vi "motor test 001.vi"() -> ()   [LabVIEW 2019]
uses:
  <vilib>/Platform/TimedLoop/XDataNode/timing_clust.ctl
  <vilib>/Platform/TimedLoop/XDataNode/nitl_modes.ctl
  <vilib>/Platform/TimedLoop/XDataNode/wakeup.ctl
  low level/motor/motor.lvclass
  <vilib>/platform/TimedLoop/XDataNode/XDataNode.xnode
  <vilib>/Platform/TimedLoop/XDataNode/XDNodeRunTimeDep.lvlib
panel:
  in  "Stop":bool
  out "error out":errorcluster
  in  "Error In":errorcluster
  in  "Vertical Pointer Slide":dbl(slide) scale=-125.0..125.0
  in  "reset":bool
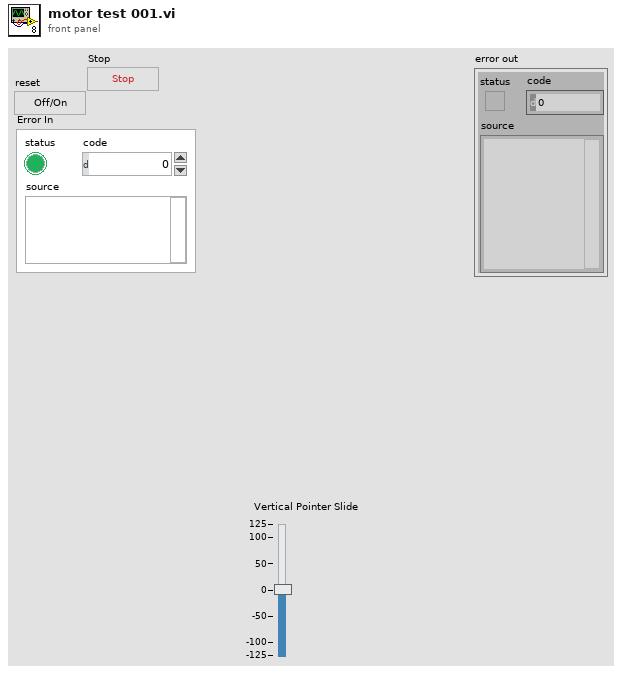
[diagram p1: front panel]
types:
  T1 = typedef "XDNodeRunTimeDep.lvlib/timing_clust.ctl" = cluster{"Expected End [f-1]":u64, "Actual End [f-1]":u64, "Finished Late? [f-1]":bool, "Expected End [i-1]":u64, "Actual End [i-1]":u64, "Finished Late? [i-1]":bool, "Expected Start [i]":u64, "Actual Start [i]":u64, "Expected Start [f]":u64, "Actual Start [f]":u64, "Source Name":string, "Structure Name":string, "Period":i64, "Deadline":i64, "Offset":i64, "Start":i64, "Priority":i32, "Timeout":i32, "Mode":T2, "Wakeup Reason":T3, "Error":errorcluster, "Source Type":string, "Secondary Source Type":string, "Global End Time":u64, "Global Start Time":u64, "Frame Duration":u64, "Iteration Duration":u64, "Assigned CPU":i32, "I/O Scan Engine Mode":u32}
  T2 = typedef "XDNodeRunTimeDep.lvlib/nitl_modes.ctl" = enum32{"No Change", "Process missed periods, maintain original phase", "Discard missed periods, maintain original phase", "Process missed periods, ignore original phase", "Discard missed periods, ignore original phase"}
  T3 = typedef "XDNodeRunTimeDep.lvlib/wakeup.ctl" = enum32{"Normal", "Aborted", "Asynchronous wakeup", "Timing source error", "Timed loop error", "Timeout"}
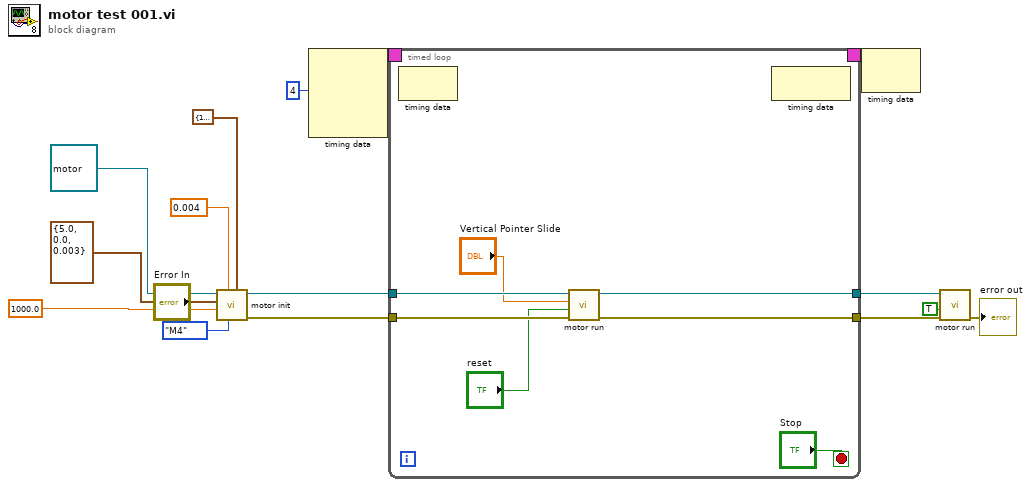
[diagram p0: block diagram]
diagram:
  n1 = call "motor init.vi"("encoder"=cluster{"encoder PPR":dbl, "gear ratio":dbl} {"encoder PPR"=16.0, "gear ratio"=64.0}, "motor  ?"=enum16{"M1", "M2", "M3", "M4"}."M4", "dt"=0.004, "Error In"="Error In", "PWM frequence"=1000.0, "PID"=cluster{"Kp":dbl, "Ki":dbl, "Kd":dbl} {"Kp"=5.0, "Ki"=0.0, "Kd"=0.003}, "class in"=refnum<class "motor.lvclass"> refnum) -> ("error out"=w12:errorcluster, "class out"=w16:refnum<class "motor.lvclass">)  [unwired: 3 in]
  n2 = node-c288(i64 4 ("Period")) -> (w15:T1)  [unwired: 3 in]
  n3 = timed-loop {
    timing: w15 -> [_]
    timing-out: [_] -> w14
    tunnel: w16 -> [w23]
    tunnel: w12 -> [w22]
    tunnel: [w19] -> w5
    tunnel: [w18] -> w4
    stop <- "Stop" stop-if-true
    n4 = node-c288() -> ()  [unwired: 1 in, 1 out]
    n5 = call-dynamic "motor run.vi"("error in (no error)"=w22, "reset"="reset", "speed"="Vertical Pointer Slide", "motor in"=w23) -> ("error out"=w19:errorcluster, "motor out"=w18:refnum<class "motor.lvclass">)  [unwired: 6 in]
    n6 = node-c288() -> ()  [unwired: 1 in, 1 out]
  }
  n7 = node-c288(w14) -> ()  [unwired: 1 out]
  n8 = call-dynamic "motor run.vi"("error in (no error)"=w5, "reset"=TRUE, "motor in"=w4) -> ("error out"=→"error out":errorcluster)  [unwired: 7 in, 1 out]
